vi "Geometry_Sample.vi"() -> ()   [LabVIEW 2019]
uses:
  SubVIs/ROBOT_PICTURE.ctl
  <vilib>/Rock Robotics/WPI/ThirdParty/JAS_Junk/TrajLib/TypeDef/POSE2D.ctl
  <vilib>/Rock Robotics/WPI/ThirdParty/JAS_Junk/TrajLib/TypeDef/TRANSLATION2D.ctl
  <vilib>/Rock Robotics/WPI/ThirdParty/JAS_Junk/TrajLib/TypeDef/ROTATION2D.ctl
  <vilib>/Rock Robotics/WPI/ThirdParty/JAS_Junk/TrajLib/Rotation2d_CreateAngle.vi
  <vilib>/Rock Robotics/WPI/ThirdParty/JAS_Junk/TrajLib/Translation2d_Create.vi
  <vilib>/Rock Robotics/WPI/ThirdParty/JAS_Junk/TrajLib/Transform2d_Create_PosePose.vi
  <vilib>/Rock Robotics/WPI/ThirdParty/JAS_Junk/TrajLib/Pose2d_New_TRRO.vi
  <vilib>/Rock Robotics/WPI/ThirdParty/JAS_Junk/TrajLib/Util_CalcDist.vi
  <vilib>/Rock Robotics/WPI/ThirdParty/JAS_Junk/TrajLib/Rotation2d_UnaryMinus.vi
  <vilib>/Rock Robotics/WPI/ThirdParty/JAS_Junk/TrajLib/Translation2d_RotateBy.vi
  <vilib>/Rock Robotics/WPI/ThirdParty/JAS_Junk/TrajLib/Translation2d_Minus.vi
  <vilib>/Rock Robotics/WPI/ThirdParty/JAS_Junk/TrajLib/Rotation2d_Minus.vi
  <vilib>/Rock Robotics/WPI/ThirdParty/JAS_Junk/TrajLib/Rotation2d_RotateBy.vi
  <vilib>/picture/pixmap.llb/Flatten Pixmap.vi
  <vilib>/picture/pictutil.llb/Create Mask.vi
  <vilib>/picture/picture.llb/Draw Flattened Pixmap.vi
  <vilib>/Rock Robotics/WPI/ThirdParty/JAS_Junk/TrajLib/Trajectory_Library.lvlib
panel:
  in  "Tab Control":enum32{"FIeld", "Additional Data"}(tab)
  out "Robot":T1
  out "BALL":bool=TRUE
  out "Robot POSE":T2 {"ROTATION"."SIN" format="%13.4f"; "ROTATION"."COS" format="%13.4f"; "ROTATION"."VALUE" format="%13.4f"; "TRANSLATION"."Y" format="%14.3f"; "TRANSLATION"."X" format="%14.3f"}
  out "Ball POSE":T2 {"ROTATION"."SIN" format="%13.4f"; "ROTATION"."COS" format="%13.4f"; "ROTATION"."VALUE" format="%13.4f"; "TRANSLATION"."Y" format="%14.3f"; "TRANSLATION"."X" format="%14.3f"}
  out "Pose Ball Relative to Robot":T2 {"ROTATION"."SIN" format="%13.4f"; "ROTATION"."COS" format="%13.4f"; "ROTATION"."VALUE" format="%13.4f"; "TRANSLATION"."Y" format="%14.3f"; "TRANSLATION"."X" format="%14.3f"}
  out "Angle To Ball (Degrees)":dbl
  out "Distance To Ball (Inches)":dbl
  in  "Y  INCHES - BALL":dbl=150.0
  in  "X INCHES - BALL":dbl=200.0
  in  "ORIENTATION - DEG":dbl=42.0
  in  "Y  INCHES":dbl=150.0
  in  "X INCHES":dbl=46.0
  # "Geometry Sample"
  # "ROBOT"
  # "BALL"
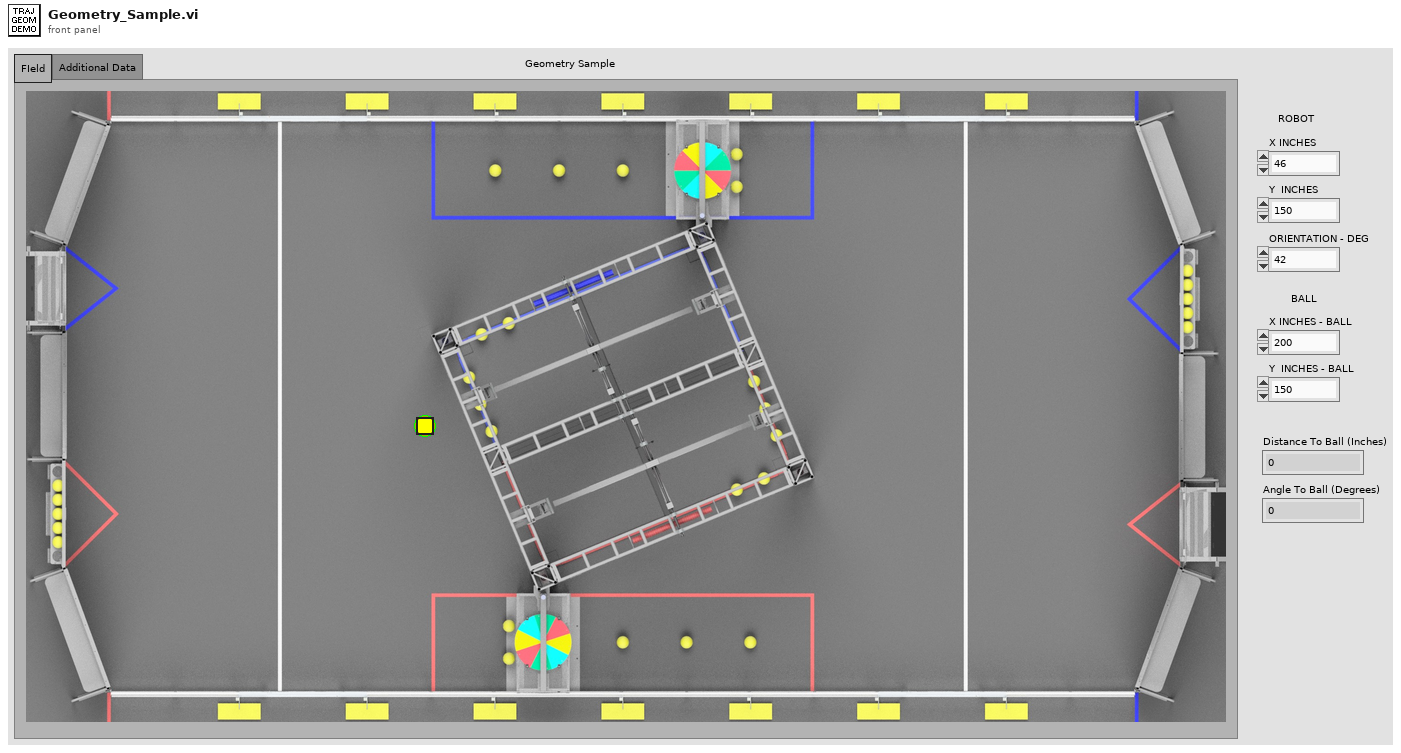
[diagram p1: front panel]
types:
  T1 = typedef "ROBOT_PICTURE.ctl" = picture
  T2 = typedef "Trajectory_Library.lvlib/POSE2D.ctl" = cluster{"TRANSLATION":T3, "ROTATION":T4}
  T3 = typedef "Trajectory_Library.lvlib/TRANSLATION2D.ctl" = cluster{"X":dbl, "Y":dbl}
  T4 = typedef "Trajectory_Library.lvlib/ROTATION2D.ctl" = cluster{"VALUE":dbl, "COS":dbl, "SIN":dbl}
  T5 = typedef "Rotated_Picture_TypeDef.ctl" = cluster{"ONE-8-bit pixmap":u8[][], "Two-Array":cdb[][], "Three-Numeric":i32, "Four-Numeric":i32, "Five-Numeric":cdb, "Six-colors":u32[], "Seven-new element/subarray":u32, "Eight-Cluster":cluster{"[0]":i32, "[1]":i32}}
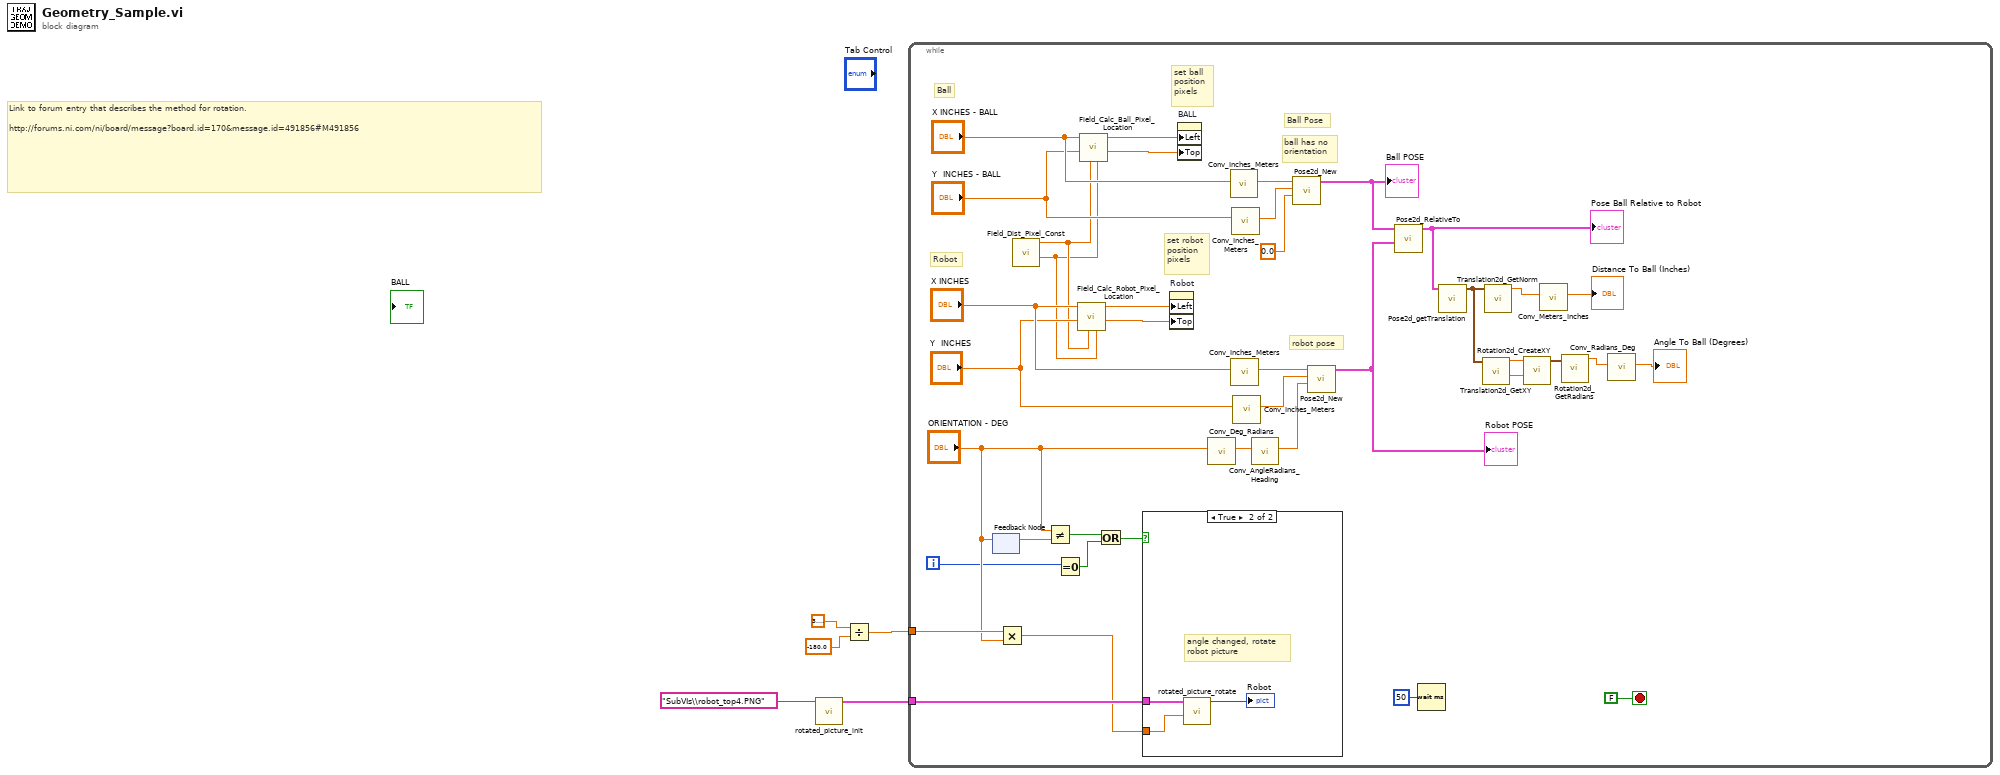
[diagram p0: block diagram]
diagram:
  # "Link to forum entry that describes the method for rotation.\n\nhttp://forums.ni.com/ni/board/message?board.id=170&message.id=491856#M491856"
  n1 = call "rotated_picture_init.vi"("Picture FIle Name"="SubVIs\\robot_top4.PNG" ("name or relative path")) -> ("RotatedPictureInfo"=w1:T5)  [unwired: 10 in]
  n2 = Divide(x=3.141592653589793, y=-180.0 ("value")) -> (x/y=w3:dbl)
  n3 = while {
    tunnel: w3 -> [w44]
    tunnel: w1 -> [w43]
    i -> [w27]
    stop <- FALSE stop-if-true
    # "Ball"
    # "Robot"
    # "ball has no\norientation"
    # "robot pose"
    # "Ball Pose"
    # "set robot\nposition\npixels"
    # "set ball \nposition\npixels"
    n4 = feedback-in #1("ORIENTATION - DEG") -> ()
    n5 = feedback #1() -> (w39:dbl)  [unwired: 1 in]
    n6 = Multiply(x=w44, y="ORIENTATION - DEG") -> (x*y=w41:dbl)
    n7 = call "Field_Dist_Pixel_Const.vi"() -> ("Y Conv"=w6:dbl, "X Conv"=w7:dbl)  [unwired: 10 in]
    n8 = Not Equal?(x="ORIENTATION - DEG", y=w39) -> (x != y?=w29:bool)
    n9 = Equal To 0?(x=w27) -> (x = 0?=w28:bool)
    n10 = call "Field_Calc_Robot_Pixel_Location.vi"("Y Conv"=w6, "X Conv"=w7, "Y  INCHES"="Y  INCHES", "X INCHES"="X INCHES") -> ("Top Pixel"=w10:dbl, "Left Pixel"=w38:dbl)  [unwired: 6 in]
    n11 = call "Field_Calc_Ball_Pixel_Location.vi"("Y Conv"=w6, "X Conv"=w7, "Y  INCHES - BALL"="Y  INCHES - BALL", "X INCHES - BALL"="X INCHES - BALL") -> ("Top Pixel"=w11:dbl, "Left Pixel"=w37:dbl)  [unwired: 6 in]
    n12 = Or(x=w29, y=w28) -> (x .or. y?=w30:bool)
    n13 = case shown="True" w30 {
      tunnel: w43 -> [_ w46]
      tunnel: w41 -> [_ w45]
      frame False {
        # "Leave as is..."
      }
      frame True {
        # "angle changed, rotate\nrobot picture"
        n14 = call "rotated_picture_rotate.vi"("Angle"=w45, "RotatedPictureInfo"=w46) -> ("new picture"=→"Robot":picture)  [unwired: 9 in]
      }
    }
    n15 = property on="Robot" class="Pict (strict)"("Left"=w38, "Top"=w10) -> ()  [unwired: 2 in, 2 out]
    n16 = property on="BALL" class="Bool (strict)"("Left"=w37, "Top"=w11) -> ()  [unwired: 2 in, 2 out]
    n17 = call <vilib>:"Conv_Deg_Radians.vi"("Degress"="ORIENTATION - DEG") -> ("Radians"=w35:dbl)  [unwired: 10 in]
    n18 = call <vilib>:"Conv_Inches_Meters.vi"("INCH"="X INCHES - BALL") -> ("Meters"=w26:dbl)  [unwired: 10 in]
    n19 = call <vilib>:"Conv_Inches_Meters.vi"("INCH"="X INCHES") -> ("Meters"=w34:dbl)  [unwired: 10 in]
    n20 = call <vilib>:"Conv_Inches_Meters.vi"("INCH"="Y  INCHES - BALL") -> ("Meters"=w25:dbl)  [unwired: 10 in]
    n21 = call <vilib>:"Conv_Inches_Meters.vi"("INCH"="Y  INCHES") -> ("Meters"=w33:dbl)  [unwired: 10 in]
    n22 = call <vilib>:"Conv_AngleRadians_Heading.vi"("Radians"=w35) -> ("Heading"=w31:dbl)  [unwired: 10 in]
    n23 = call <vilib>:"Pose2d_New.vi"("Heading"=0.0 ("x"), "Y"=w25, "X"=w26) -> ("out POSe"=w22:T2)  [unwired: 8 in]
    "Ball POSE" <- w22
    n24 = call <vilib>:"Pose2d_New.vi"("Heading"=w31, "Y"=w33, "X"=w34) -> ("out POSe"=w21:T2)  [unwired: 8 in]
    "Robot POSE" <- w21
    n25 = call <vilib>:"Pose2d_RelativeTo.vi"("other POSE"=w21, "in POSE"=w22) -> ("out POSE"=w23:T2)  [unwired: 9 in]
    "Pose Ball Relative to Robot" <- w23
    n26 = Wait (ms)(milliseconds to wait=u32 50) -> ()  [unwired: 1 out]
    n27 = call <vilib>:"Pose2d_getTranslation.vi"("in POSE"=w23) -> ("outTRANSLATION"=w20:T3)  [unwired: 10 in]
    n28 = call <vilib>:"Translation2d_GetXY.vi"("In Translation"=w20) -> ("Y"=w18:dbl, "X"=w19:dbl)  [unwired: 9 in]
    n29 = call <vilib>:"Translation2d_GetNorm.vi"("In Translation"=w20) -> ("Norm"=w14:dbl)  [unwired: 10 in]
    n30 = call <vilib>:"Rotation2d_CreateXY.vi"("Y or sine"=w18, "X or  cosine"=w19) -> ("ROTATION"=w17:T4)  [unwired: 9 in]
    n31 = call <vilib>:"Conv_Meters_Inches.vi"("Meters"=w14) -> ("Inches"=→"Distance To Ball (Inches)":dbl)  [unwired: 10 in]
    n32 = call <vilib>:"Rotation2d_GetRadians.vi"("in ROTATION"=w17) -> ("AngleRadians"=w16:dbl)  [unwired: 10 in]
    n33 = call <vilib>:"Conv_Radians_Deg.vi"("Radians"=w16) -> ("Degrees"=→"Angle To Ball (Degrees)":dbl)  [unwired: 10 in]
  }
